vi "golpi_mpc_close_session.vi"(8 "error in":errorcluster, 10 "exit octave (true)":bool=TRUE, 11 "golpi session ref":T1) -> (0 "error out":errorcluster, 3 "golpi session ref out (copy)":T1)   [LabVIEW 2013, in "GOLPI Multi Process.lvlib"]
doc: "Close multi-process GOLPI session. Call this as a last function when you no longer need to use GOLPI via the multi-process functions. Deletes exclusive access semaphore. By default also closes GOLPI (Octave) and before the exit it executes 'exit command' stored in the GOLPI session. This is handy for instance for automatic storate of Octave environment variables."
uses:
  GOLPI Multi Process.lvlib
  golpi_session_ref.ctl
  golpi_session.ctl
  GOLPI Library.lvlibp/Public/GOLPI reference Type Def.ctl
  GOLPI Library.lvlibp/LV Process source distribution/Pipe Handle.ctl
  GOLPI Library.lvlibp/LV Process source distribution/LV Process library.lvlib
  GOLPI Library.lvlibp
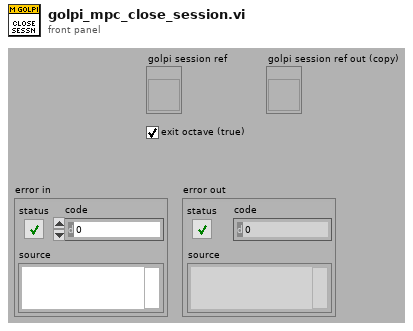
[diagram p1: front panel]
types:
  T1 = typedef "GOLPI Multi Process.lvlib/golpi_session_ref.ctl" = refnum<vi>
  T2 = typedef "Semaphore RefNum" = refnum<k1>
  T3 = typedef "GOLPI Multi Process.lvlib/golpi_session.ctl" = cluster{"GOLPI ref":T4, "idn str":string, "octave path":path, "work path":path, "start timeout [ms]":u32, "clr cache":bool, "console":bool, "binary":bool, "semaphore":T2, "initial command":string, "exit command":string, "matlab":bool}
  T4 = typedef "GOLPI Library.lvlibp/GOLPI reference Type Def.ctl" = cluster{"pipe handle":T5, "fast read timeout [ms]":u32, "fast read settle time [ms]":u32, "fast read to multiple [ms]":u32, "max elements per input line":u32, "slow read timeout [ms]":u32, "stdin double format specifier":string, "max elements per stdout output column":u32, "console mode bitstream":bool, "bitstream first read timeout [ms]":u32, "bitstream read timeout [ms]":u32, "struct transfer possible":bool, "matlab mode":bool}
  T5 = typedef "GOLPI Library.lvlibp/LV Process library.lvlib/Pipe Handle.ctl" = cluster{"lv_proc.dll file path":path, "process instance handle":u32[], "debug mode":bool, "debug data":cluster{"time":timestamp, "stdin":bool, "data":string}[]}
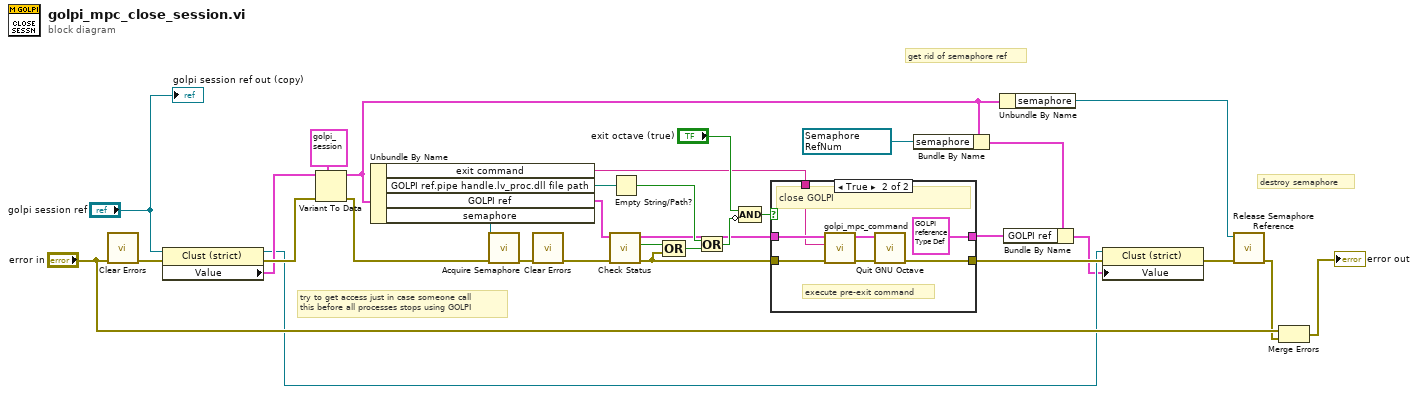
[diagram p0: block diagram]
diagram:
  w29 = T2 refnum items=["semaphore"] ("semaphore")
  # "destroy semaphore"
  # "get rid of semaphore ref"
  # "try to get access just in case someone call\nthis before all processes stops using GOLPI"
  n1 = call <vilib>:"Clear Errors.vi"("error in (no error)"="error in") -> ("error out"=w25:errorcluster)  [unwired: 6 in]
  n2 = property class="Clust (strict)"(reference="golpi session ref", error in=w25) -> (reference out=w18:T1, error out=w32:errorcluster, "Value"=w31:T3)
  n3 = Variant To Data(error in=w32, type=T3 {"GOLPI ref"={"pipe handle"={"lv_proc.dll file path"=path "", "process instance handle"=[], "debug mode"=FALSE, "debug data"=[]}, "fast read timeout [ms]"=0, "fast read settle time [ms]"=0, "fast read to multiple [ms]"=0, "max elements per input line"=0, "slow read timeout [ms]"=0, "stdin double format specifier"="", "max elements per stdout output column"=0, "console mode bitstream"=FALSE, "bitstream first read timeout [ms]"=0, "bitstream read timeout [ms]"=0, "struct transfer possible"=FALSE, "matlab mode"=FALSE}, "idn str"="", "octave path"=path "", "work path"=path "", "start timeout [ms]"=0, "clr cache"=FALSE, "console"=FALSE, "binary"=FALSE, "semaphore"=refnum, "initial command"="", "exit command"="", "matlab"=FALSE} ("golpi session"), Variant=w31) -> (data=w2:T3, error out=w19:errorcluster)
  n4 = Unbundle By Name(w2) -> ("exit command"=w5:string, "GOLPI ref.pipe handle.lv_proc.dll file path"=w12:path, "GOLPI ref"=w15:T4, "semaphore"=w20:T2)
  n5 = call <vilib>:"Acquire Semaphore.vi"("error in (no error)"=w19, "semaphore"=w20) -> ("error out"=w17:errorcluster)  [unwired: 3 in, 2 out]
  n6 = call <vilib>:"Clear Errors.vi"("error in (no error)"=w17) -> ("error out"=w16:errorcluster)  [unwired: 6 in]
  n7 = call "Check Status.vi"("error in"=w16, "GOLPI ref. in"=w15) -> ("error out"=w6:errorcluster, "exited?"=w11:bool, "GOLPI ref. out"=w7:T4)  [unwired: 7 in]
  n8 = Empty String/Path?(string/path=w12) -> (empty?=w13:bool)
  n9 = Compound Arithmetic op=OR(w11, w6) -> (w14:bool)
  n10 = Or(x=w13, y=w14) -> (x .or. y?=w10:bool)
  n11 = Compound Arithmetic op=AND("exit octave (true)", invert w10) -> (w8:bool)
  n12 = case shown="True" w8 {
    tunnel: [w34 w39] -> w23
    tunnel: w6 -> [w34 w37]
    tunnel: [w33 T4 {"pipe handle"={"lv_proc.dll file path"=path "", "process instance handle"=[], "debug mode"=FALSE, "debug data"=[]}, "fast read timeout [ms]"=0, "fast read settle time [ms]"=0, "fast read to multiple [ms]"=0, "max elements per input line"=0, "slow read timeout [ms]"=0, "stdin double format specifier"="", "max elements per stdout output column"=0, "console mode bitstream"=FALSE, "bitstream first read timeout [ms]"=0, "bitstream read timeout [ms]"=0, "struct transfer possible"=FALSE, "matlab mode"=FALSE} ("GOLPI ref")] -> w3
    tunnel: w7 -> [w33 w38]
    tunnel: w5 -> [_ w36]
    frame False {
    }
    frame True {
      # "execute pre-exit command"
      # "close GOLPI"
      n13 = call "golpi_mpc_command.vi"("error in"=w37, "command"=w36, "GOLPI ref in"=w38) -> ("error out"=w40:errorcluster, "GOLPI ref. out"=w41:T4)  [unwired: 6 in, 1 out]
      n14 = call "Quit GNU Octave.vi"("error in"=w40, "GOLPI ref. in"=w41) -> ("error out"=w39:errorcluster)  [unwired: 8 in, 1 out]
    }
  }
  n15 = Bundle By Name(cluster=w2, "semaphore"=w29) -> (w4:T3)
  n16 = Unbundle By Name(w2) -> ("semaphore"=w27:T2)
  n17 = Bundle By Name(cluster=w4, "GOLPI ref"=w3) -> (w1:T3)
  n18 = property class="Clust (strict)"(reference=w18, error in=w23, "Value"=w1) -> (error out=w28:errorcluster)  [unwired: 1 out]
  n19 = call <vilib>:"Release Semaphore Reference.vi"("error in (no error)"=w28, "semaphore"=w27) -> ("error out"=w24:errorcluster)  [unwired: 8 in, 1 out]
  n20 = Merge Errors("error in", w24) -> (→"error out":errorcluster)
  "golpi session ref out (copy)" <- "golpi session ref"
